vi "SP Check for Stimulus Change.vi"(6 "Current Stimulus Channel":T1={"Use Instrument Settings"=FALSE, "Blank Frequencies"=FALSE, "Sweep Type"=enum."Linear", "Sweep"={"Fstart"=500.0, "Fstop"=1500.0, "Units"=enum."MHz", "Points"=201}, "Power (dBm)"=999.0, "IFBW (Hz)"=-1.0, "Sweep Time (s)"=-1.0, "Calibration"={"State"=FALSE, "String"=""}} {"Sweep Time (s)" format="%.3g"}, 10 "Current Stimulus In":T1={"Use Instrument Settings"=FALSE, "Blank Frequencies"=FALSE, "Sweep Type"=enum."Linear", "Sweep"={"Fstart"=500.0, "Fstop"=1500.0, "Units"=enum."MHz", "Points"=201}, "Power (dBm)"=999.0, "IFBW (Hz)"=-1.0, "Sweep Time (s)"=-1.0, "Calibration"={"State"=FALSE, "String"=""}} {"Sweep Time (s)" format="%.3g"}, 11 "New Stimulus":T1={"Use Instrument Settings"=FALSE, "Blank Frequencies"=FALSE, "Sweep Type"=enum."Linear", "Sweep"={"Fstart"=500.0, "Fstop"=1500.0, "Units"=enum."MHz", "Points"=201}, "Power (dBm)"=999.0, "IFBW (Hz)"=-1.0, "Sweep Time (s)"=-1.0, "Calibration"={"State"=FALSE, "String"=""}} {"Sweep Time (s)" format="%.3g"}) -> (1 "Stimulus Changed?":bool, 2 "Current Stimulus Out":T1={"Use Instrument Settings"=FALSE, "Blank Frequencies"=FALSE, "Sweep Type"=enum."Linear", "Sweep"={"Fstart"=500.0, "Fstop"=1500.0, "Units"=enum."MHz", "Points"=201}, "Power (dBm)"=999.0, "IFBW (Hz)"=-1.0, "Sweep Time (s)"=-1.0, "Calibration"={"State"=FALSE, "String"=""}} {"Sweep Time (s)" format="%.3g"}, 3 "Stimulus to Set":T1={"Use Instrument Settings"=FALSE, "Blank Frequencies"=FALSE, "Sweep Type"=enum."Linear", "Sweep"={"Fstart"=500.0, "Fstop"=1500.0, "Units"=enum."MHz", "Points"=201}, "Power (dBm)"=999.0, "IFBW (Hz)"=-1.0, "Sweep Time (s)"=-1.0, "Calibration"={"State"=FALSE, "String"=""}} {"Sweep Time (s)" format="%.3g"})   [LabVIEW 2011]
uses:
  TypeDefs/SP Stimulus Parameters.ctl
  TypeDefs/SP Frequency Units.ctl
  TypeDefs/SP Calibration State.ctl
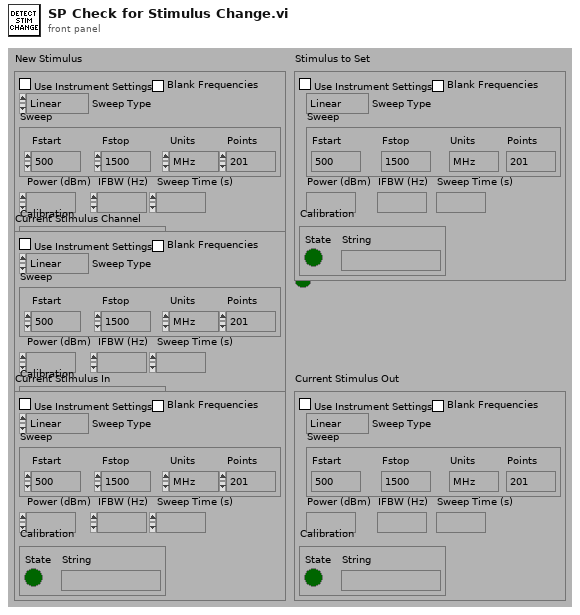
[diagram p1: front panel]
types:
  T1 = typedef "SP Stimulus Parameters.ctl" = cluster{"Use Instrument Settings":bool, "Blank Frequencies":bool, "Sweep Type":enum32{"Linear", "Logarithmic", "List", "Power", "CW"}, "Sweep":cluster{"Fstart":dbl, "Fstop":dbl, "Units":T2, "Points":i32}, "Power (dBm)":dbl, "IFBW (Hz)":dbl, "Sweep Time (s)":dbl, "Calibration":T3}
  T2 = typedef "SP Frequency Units.ctl" = enum16{"Hz", "kHz", "MHz", "GHz", "Points"}
  T3 = typedef "SP Calibration State.ctl" = cluster{"State":bool, "String":string}
  T4 = enum32{"Linear", "Logarithmic", "List", "Power", "CW"}
  T5 = cluster{"Fstart":dbl, "Fstop":dbl, "Units":T2, "Points":i32}
  T6 = cluster{"Converted Frequency":dbl, "Converted Frequency":dbl, "Points":i32, "Sweep Type":enum32{"Linear", "Logarithmic", "List", "Power", "CW"}}
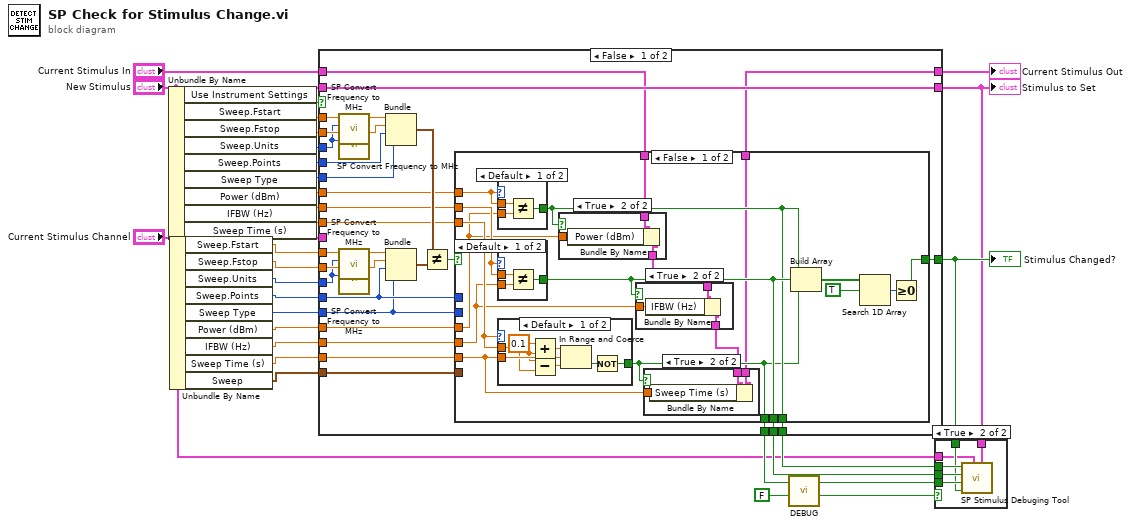
[diagram p0: block diagram]
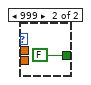
[diagram p6: hidden frame]
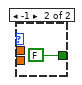
[diagram p7: hidden frame]
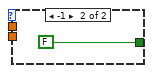
[diagram p8: hidden frame]
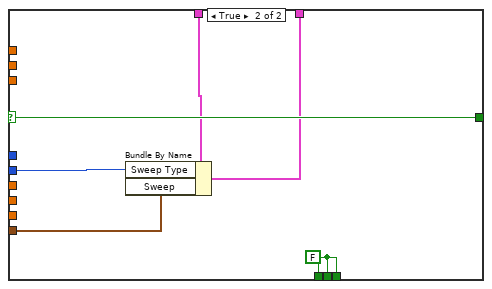
[diagram p9: hidden frame]
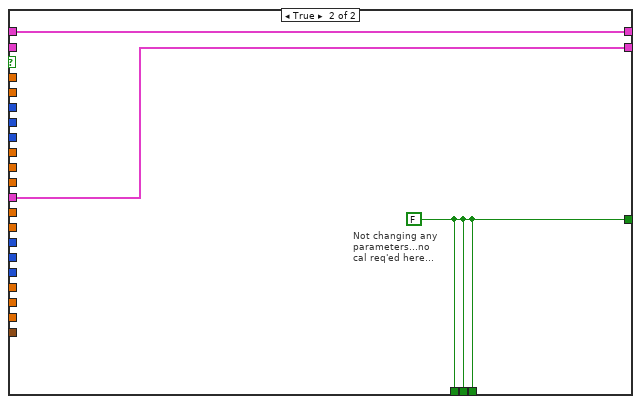
[diagram p10: hidden frame]
diagram:
  n1 = Unbundle By Name("New Stimulus") -> ("Use Instrument Settings"=w29:bool, "Sweep.Fstart"=w7:dbl, "Sweep.Fstop"=w6:dbl, "Sweep.Units"=w5:T2, "Sweep.Points"=w26:i32, "Sweep Type"=w28:T4, "Power (dBm)"=w24:dbl, "IFBW (Hz)"=w22:dbl, "Sweep Time (s)"=w20:dbl)
  n2 = Unbundle By Name("Current Stimulus Channel") -> ("Sweep.Fstart"=w4:dbl, "Sweep.Fstop"=w3:dbl, "Sweep.Units"=w2:T2, "Sweep.Points"=w25:i32, "Sweep Type"=w27:T4, "Power (dBm)"=w23:dbl, "IFBW (Hz)"=w21:dbl, "Sweep Time (s)"=w19:dbl, "Sweep"=w1:T5)
  n3 = case shown="False" w29 {
    tunnel: w25 -> [w43 _]
    tunnel: w23 -> [w50 _]
    tunnel: w21 -> [w49 _]
    tunnel: w26 -> [w60 _]
    tunnel: w24 -> [w53 _]
    tunnel: w22 -> [w52 _]
    tunnel: "New Stimulus" -> [w57 _]
    tunnel: "Current Stimulus Channel" -> [_ w114]
    tunnel: [w57 w114] -> w12
    tunnel: [w54 w113] -> w15
    tunnel: w19 -> [w48 _]
    tunnel: w20 -> [w51 _]
    tunnel: w28 -> [w56 _]
    tunnel: w27 -> [w42 _]
    tunnel: [w47 w113] -> w18
    tunnel: [w46 w113] -> w17
    tunnel: [w45 w113] -> w16
    tunnel: "Current Stimulus In" -> [w44 w112]
    tunnel: [w41 w112] -> w8
    tunnel: w7 -> [w40 _]
    tunnel: w6 -> [w37 _]
    tunnel: w5 -> [w35 _]
    tunnel: w4 -> [w39 _]
    tunnel: w3 -> [w38 _]
    tunnel: w2 -> [w36 _]
    tunnel: w1 -> [w30 _]
    frame False {
      n4 = call "SP Convert Frequency to MHz.vi"("Units"=w35, "Frequency"=w40) -> ("Converted Frequency"=w34:dbl)  [unwired: 1 in, 8 out]
      n5 = call "SP Convert Frequency to MHz.vi"("Units"=w35, "Frequency"=w37) -> ("Converted Frequency"=w33:dbl)  [unwired: 1 in, 8 out]
      n6 = call "SP Convert Frequency to MHz.vi"("Units"=w36, "Frequency"=w39) -> ("Converted Frequency"=w31:dbl)  [unwired: 1 in, 8 out]
      n7 = call "SP Convert Frequency to MHz.vi"("Units"=w36, "Frequency"=w38) -> ("Converted Frequency"=w32:dbl)  [unwired: 1 in, 8 out]
      n8 = Bundle("Converted Frequency"=w34, "Converted Frequency"=w33, "Points"=w60, "Sweep Type"=w56) -> (w58:T6)  [unwired: 1 out]
      n9 = Bundle("Converted Frequency"=w31, "Converted Frequency"=w32, "Points"=w43, "Sweep Type"=w42) -> (w59:T6)  [unwired: 1 out]
      n10 = Not Equal?(x=w58, y=w59) -> (x != y?=w55:bool)
      n11 = case shown="False" w55 {
        selector: w55 -> [_ w111]
        tunnel: [w71 w111] -> w54
        tunnel: w53 -> [w75 _]
        tunnel: w52 -> [w76 _]
        tunnel: w51 -> [w77 _]
        tunnel: w50 -> [w69 _]
        tunnel: w49 -> [w67 _]
        tunnel: w48 -> [w63 _]
        tunnel: [w65 w110] -> w47
        tunnel: [w68 w110] -> w46
        tunnel: [w64 w110] -> w45
        tunnel: w44 -> [w70 w109]
        tunnel: w43 -> [_ _]
        tunnel: w42 -> [_ w108]
        tunnel: [w61 w107] -> w41
        tunnel: w30 -> [_ w106]
        frame False {
          n12 = case shown="Default" w75 {
            tunnel: w75 -> [w92 _]
            tunnel: w69 -> [w91 _]
            tunnel: [w90 FALSE] -> w65
            frame Default {
              n13 = Not Equal?(x=w92, y=w91) -> (x != y?=w90:bool)
            }
            frame 999 {
            }
          }
          n14 = case shown="Default" w76 {
            tunnel: w76 -> [w96 _]
            tunnel: w67 -> [w95 _]
            tunnel: [w94 FALSE] -> w68
            frame Default {
              n15 = Not Equal?(x=w96, y=w95) -> (x != y?=w94:bool)
            }
            frame -1 {
            }
          }
          n16 = case shown="Default" w77 {
            tunnel: w77 -> [w98 _]
            tunnel: w63 -> [w102 _]
            tunnel: [w99 FALSE] -> w64
            frame Default {
              w100 = 0.1
              n17 = Add(x=w100, y=w98) -> (x+y=w103:dbl)
              n18 = Subtract(x=w98, y=w100) -> (x-y=w101:dbl)
              n19 = In Range and Coerce(upper limit=w103, x=w102, lower limit=w101) -> (In Range?=w104:bool)  [unwired: 1 out]
              n20 = Not(x=w104) -> (.not. x?=w99:bool)
            }
            frame -1 {
            }
          }
          n21 = case shown="True" w65 {
            tunnel: w69 -> [_ w89]
            tunnel: w70 -> [w86 w88]
            tunnel: [w86 w87] -> w66
            frame False {
            }
            frame True {
              n22 = Bundle By Name(cluster=w88, "Power (dBm)"=w89) -> (w87:T1)
            }
          }
          n23 = case shown="True" w68 {
            tunnel: w67 -> [_ w85]
            tunnel: w66 -> [w82 w84]
            tunnel: [w82 w83] -> w62
            frame False {
            }
            frame True {
              n24 = Bundle By Name(cluster=w84, "IFBW (Hz)"=w85) -> (w83:T1)
            }
          }
          n25 = case shown="True" w64 {
            tunnel: w63 -> [_ w81]
            tunnel: w62 -> [w78 w80]
            tunnel: [w78 w79] -> w61
            frame False {
            }
            frame True {
              n26 = Bundle By Name(cluster=w80, "Sweep Time (s)"=w81) -> (w79:T1)
            }
          }
          n27 = Build Array(w65, w68, w64) -> (w74:bool[])
          n28 = Search 1D Array(1D array=w74, element=TRUE) -> (index of element=w72:i32)  [unwired: 1 out]
          n29 = Greater Or Equal To 0?(x=w72) -> (x >= 0?=w71:bool)
        }
        frame True {
          w110 = FALSE
          n30 = Bundle By Name(cluster=w109, "Sweep Type"=w108, "Sweep"=w106) -> (w107:T1)
        }
      }
    }
    frame True {
      w113 = FALSE
      # "Not changing any\nparameters...no\ncal req'ed here..."
    }
  }
  "Stimulus Changed?" <- w15
  "Stimulus to Set" <- w12
  "Current Stimulus Out" <- w8
  n31 = call "DEBUG.vi"("Dev DEBUG? (f)"=FALSE) -> ("DEBUG?"=w11:bool)  [unwired: 1 in, 5 out]
  n32 = case shown="True" w11 {
    tunnel: w18 -> [_ w120]
    tunnel: w17 -> [_ w119]
    tunnel: w16 -> [_ w118]
    tunnel: w15 -> [_ w117]
    tunnel: "Current Stimulus Channel" -> [_ w116]
    tunnel: w12 -> [_ w115]
    frame False {
    }
    frame True {
      n33 = call "SP Stimulus Debuging Tool.vi"("New Stimulus"=w115, "Current Stimulus"=w116, "Overall"=w117, "SweepTime"=w118, "IFBW"=w119, "Power"=w120) -> ()  [unwired: 6 out]
    }
  }
